vi "UpdateStack.vi"(4 "Contrast":dbl=1.0, 5 "Scan Settings":T1, 6 "Offset":dbl, 8 "Section":u32, 9 "ImData":i32[][](array[numeric]), 10 "Im2 2":T2, 11 "Im1 In":T2) -> (2 "Im2 Out":T2, 3 "Im1 Out":T2)   [LabVIEW 2014]
uses:
  <vilib>/vision/Image Controls.llb/IMAQ Image.ctl
  <vilib>/gmath/statdist.llb/st_Percentiles (scalar).vi
  <vilib>/gmath/NI_Gmath.lvlib
panel:
  out "size(s)":i32[](array[numeric])
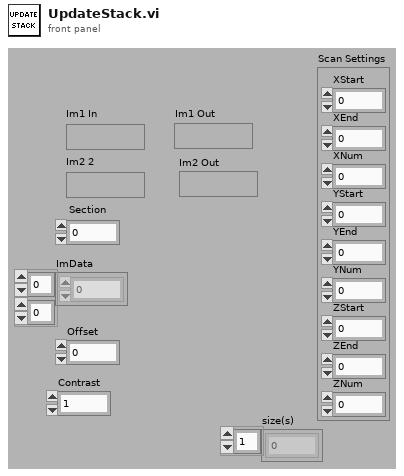
[diagram p1: front panel]
types:
  T1 = cluster{"XStart":i32, "XEnd":i32, "XNum":i32, "YStart":i32, "YEnd":i32, "YNum":i32, "ZStart":i32, "ZEnd":i32, "ZNum":i32}
  T2 = typedef "IMAQ Image.ctl" = refnum<image>
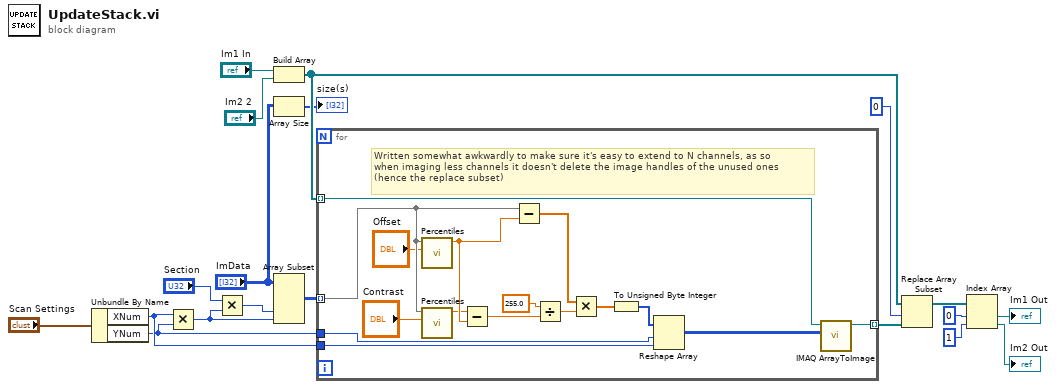
[diagram p0: block diagram]
diagram:
  n1 = Unbundle By Name("Scan Settings") -> ("XNum"=w7:i32, "YNum"=w6:i32)
  n2 = Multiply(x=w7, y=w6) -> (x*y=w3:i32)
  n3 = Multiply(x="Section", y=w3) -> (x*y=w2:u32)
  n4 = Build Array("Im1 In", "Im2 2") -> (w17:T2[])
  n5 = Array Size(array="ImData") -> (size(s)=→"size(s)":i32[])
  n6 = Array Subset(array="ImData", index (col)=w2, length (col)=w3) -> (w1:i32[][])  [unwired: 2 in]
  n7 = for {
    tunnel: w17 -> [w35] mode=indexing
    tunnel: [w34] -> w16 mode=indexing
    tunnel: w7 -> [w33]
    tunnel: w6 -> [w32]
    tunnel: w1 -> [w27] mode=indexing
    # "Written somewhat awkwardly to make sure it's easy to extend to N channels, as so\nwhen imaging less channels it doesn't delete the image handles of the unused ones\n(hence the replace subset)"
    n8 = call-poly <vilib>:"Percentiles.vi"("p"="Offset", "x array"=w27) -> ("percentile"=w26:dbl)  [unwired: 8 in, 1 out]
    n9 = call-poly <vilib>:"Percentiles.vi"("p"="Contrast", "x array"=w27) -> ("percentile"=w25:dbl)  [unwired: 8 in, 1 out]
    n10 = Subtract(x=w25, y=w26) -> (x-y=w24:dbl)
    n11 = Subtract(x=w27, y=w26) -> (x-y=w31:dbl[])
    n12 = Divide(x=255.0, y=w24) -> (x/y=w22:dbl)
    n13 = Multiply(x=w31, y=w22) -> (x*y=w30:dbl[])
    n14 = To Unsigned Byte Integer(number=w30) -> (unsigned 8bit integer=w29:u8[])
    n15 = Reshape Array(w29, w32, w33) -> (w28:u8[][])
    n16 = call "IMAQ ArrayToImage"("Image Pixels (U8)"=w28, "Image"=w35) -> ("Image Out"=w34:T2)  [unwired: 8 in, 1 out]
  }
  n17 = Replace Array Subset(array=w17, new element=w16, index=0) -> (w14:T2[])
  n18 = Index Array(array=w14, index #1=0 ("index"), index #2=1 ("index")) -> (element #1=→"Im1 Out":T2, element #2=→"Im2 Out":T2)
